vi "Read Next Message Phaeron.vi"(0 "message queue in":T3, 1 "ignore error on termination message (F)":bool, 2 "Exit? (F)":bool, 7 "termination list ([Exit])":string[](array[string])=["Exit"], 9 "timeout (1 ms)":i32=1, 11 "error in":errorcluster) -> (3 "exit process?":bool, 4 "message queue out":T3, 6 "message name":string, 8 "message value":string, 10 "timed out?":bool, 13 "acknowledge":bool, 14 "message":T1, 15 "error out":errorcluster)   [LabVIEW 2011]
doc: "Returns the next message from the message queue passed in. If the returned message matches any of the message names listed in \"termination list\" the \"exit process?\" indicator will return True."
uses:
  <vilib>/NI/AMC/AMC.lvlib
  <vilib>/NI/AMC/Message.ctl
  <vilib>/NI/AMC/Message Queue.ctl
  <vilib>/NI/Tools/Keyed Array/KeyedArray.ctl
  <vilib>/NI/Tools/Keyed Array/Tools_KeyedArray.lvlib
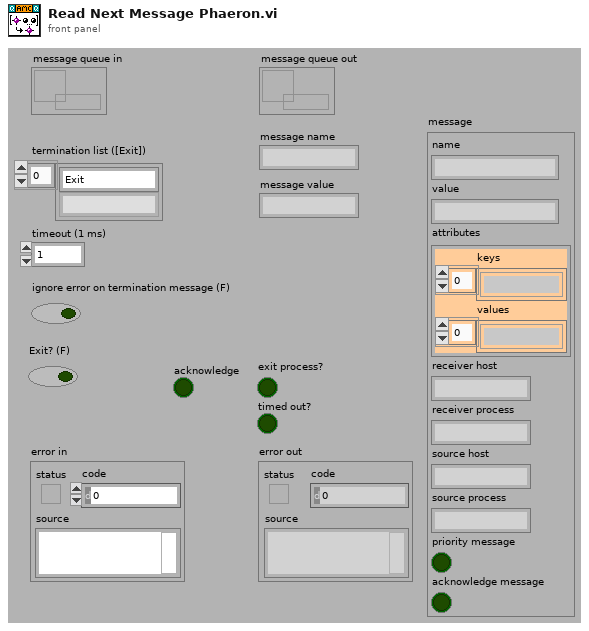
[diagram p1: front panel]
types:
  T1 = typedef "AMC.lvlib/Message.ctl" = cluster{"name":string, "value":string, "attributes":T2, "receiver host":string, "receiver process":string, "source host":string, "source process":string, "priority message":bool, "acknowledge message":bool}
  T2 = typedef "Tools_KeyedArray.lvlib/KeyedArray.ctl" = cluster{"keys":string[], "values":string[]}
  T3 = typedef "AMC.lvlib/Message Queue.ctl" = refnum<queue>
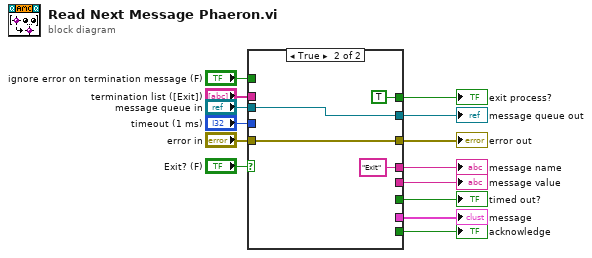
[diagram p0: block diagram]
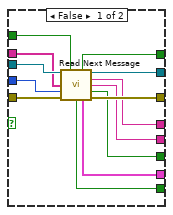
[diagram p2: hidden frame]
diagram:
  n1 = case shown="True" "Exit? (F)" {
    tunnel: "message queue in" -> [w27 w31]
    tunnel: [w22 w31] -> w12
    tunnel: "timeout (1 ms)" -> [w25 _]
    tunnel: [w15 _] -> w10
    tunnel: "termination list ([Exit])" -> [w26 _]
    tunnel: [w18 TRUE] -> w9
    tunnel: [w23 w29] -> w13
    tunnel: "error in" -> [w24 w29]
    tunnel: [w19 _] -> w4
    tunnel: [w20 _] -> w11
    tunnel: [w21 "Exit" ("name")] -> w14
    tunnel: [w16 _] -> w3
    tunnel: "ignore error on termination message (F)" -> [w17 _]
    frame False {
      n2 = call <vilib>:"Read Next Message.vi"("message queue in"=w27, "ignore error on termination message (F)"=w17, "termination list ([Exit])"=w26, "timeout (1 ms)"=w25, "error in"=w24) -> ("exit process?"=w18:bool, "message queue out"=w22:T3, "message name"=w21:string, "message value"=w20:string, "timed out?"=w19:bool, "acknowledge"=w16:bool, "message"=w15:T1, "error out"=w23:errorcluster)  [unwired: 3 in]
    }
    frame True {
    }
  }
  "message queue out" <- w12
  "message name" <- w14
  "error out" <- w13
  "message value" <- w11
  "message" <- w10
  "exit process?" <- w9
  "timed out?" <- w4
  "acknowledge" <- w3
